vi "Get Copilot Errors.vi"() -> (0 "Errors Pressent?":bool, 3 "Error Out":errorcluster)   [LabVIEW 2014]
doc: "Dequeues errors for processing\n\nThis VI will block untill an error appears in the Copilot queue."
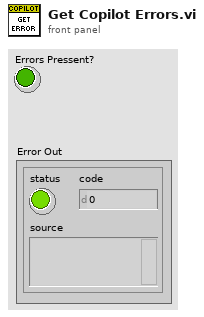
[diagram p1: front panel]
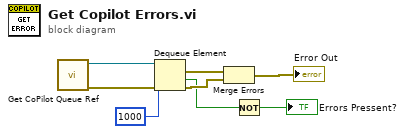
[diagram p0: block diagram]
diagram:
  n1 = call "Get CoPilot Queue Ref.vi"() -> ("Error Out"=w7:errorcluster, "queue out"=w8:refnum<queue>)  [unwired: 10 in]
  n2 = Dequeue Element(queue=w8, timeout in ms (-1)=1000, error in (no error)=w7) -> (element=w6:errorcluster, timed out?=w2:bool, error out=w5:errorcluster)  [unwired: 1 out]
  n3 = Merge Errors(w6, w5) -> (→"Error Out":errorcluster)
  n4 = Not(x=w2) -> (.not. x?=→"Errors Pressent?":bool)
